vi "Merge Error.vi"(10 "Error":errorcluster, 11 "jettl Queue Actor in":refnum<class "jettl Queue Actor.lvclass">) -> (3 "jettl Queue Actor out":refnum<class "jettl Queue Actor.lvclass">)   [LabVIEW 2021, in "jettl Queue Actor.lvlib" / "jettl Queue Actor.lvclass"]
uses:
  jettl Queue Actor.lvclass
  jettl Queue Actor.lvclass/jettl Queue Actor.ctl
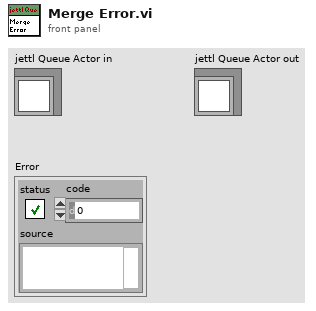
[diagram p1: front panel]
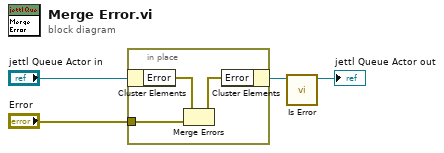
[diagram p0: block diagram]
diagram:
  n1 = in-place {
    in-place-border: "Error" -> [w5]
    n2 = in-place-cluster #1("jettl Queue Actor in") -> ("Error"=w7:errorcluster)
    n3 = Merge Errors(w7, w5) -> (w6:errorcluster)
    n4 = in-place-cluster #1("Error"=w6) -> (w2:refnum<class "jettl Queue Actor.lvclass">)
  }
  n5 = call "Is Error.vi"("jettl Queue Actor in"=w2) -> ("jettl Queue Actor out"=→"jettl Queue Actor out":refnum<class "jettl Queue Actor.lvclass">)  [unwired: 10 in]
